vi "scalarProduct.vi"(1 "amplitude matrix 2":cdb[][](array[numeric]) format="%.2f", 2 "amplitude matrix 1":cdb[][](array[numeric]) format="%.2f") -> (0 "scalar product":cdb format="%.2f")   [LabVIEW 2024]
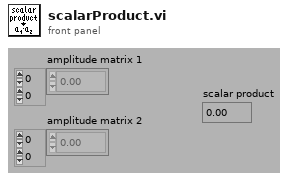
[diagram p1: front panel]
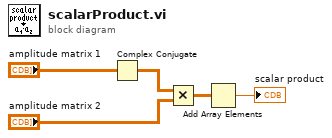
[diagram p0: block diagram]
diagram:
  n1 = Complex Conjugate(1:"amplitude matrix 1") -> (0:w4:cdb[][])
  n2 = Multiply(x=w4, y="amplitude matrix 2") -> (x*y=w2:cdb[][])
  n3 = Add Array Elements(numeric array=w2) -> (sum=→"scalar product":cdb)
